vi "图片切换.vi"() -> ()   [LabVIEW 2018]
panel:
  in  "播放速度":dbl(knob) scale=0.0..100000.0
  in  "停止":bool
  out "马里奥":u16(ring)
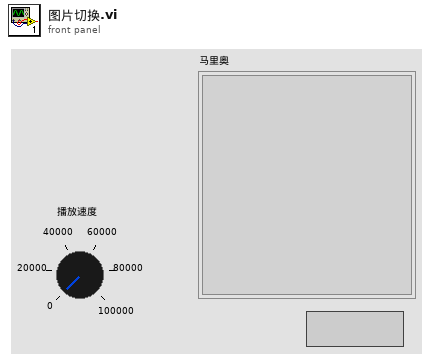
[diagram p1: front panel]
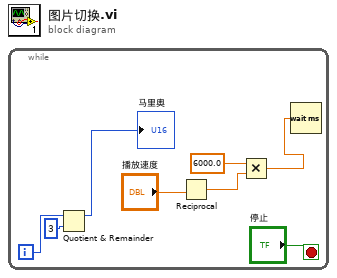
[diagram p0: block diagram]
diagram:
  n1 = while {
    i -> [w8]
    stop <- "停止" stop-if-true
    n2 = Quotient & Remainder(x=w8, y=3) -> (x-y*floor(x/y)=→"马里奥":i32)  [unwired: 1 out]
    n3 = Reciprocal(x="播放速度") -> (1/x=w3:dbl)
    n4 = Multiply(x=6000.0, y=w3) -> (x*y=w1:dbl)
    n5 = Wait (ms)(milliseconds to wait=w1) -> ()  [unwired: 1 out]
  }
